vi "context.vi"(8 "error in (no error)":errorcluster) -> (0 "error out":errorcluster, 3 "Context Out":refnum<class "Context.lvclass">)   [LabVIEW 2019, in "Context.lvclass"]
doc: "This is a constructor VI, which builds, configures and returns a context to the calling code."
uses:
  Context.lvclass
  OOP States/Initialize References/Initialize References.lvclass
  C:/Users/fflores/Documents/GitHub Projects/Simon/Simon Game/OOP States/State/State.lvclass
  ContextData/ContextData.lvclass
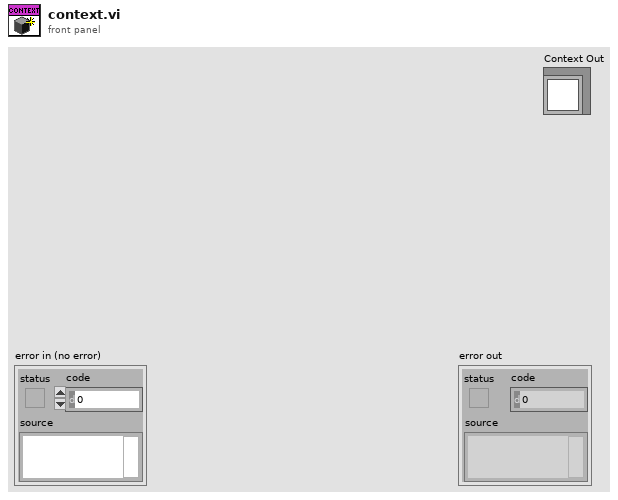
[diagram p1: front panel]
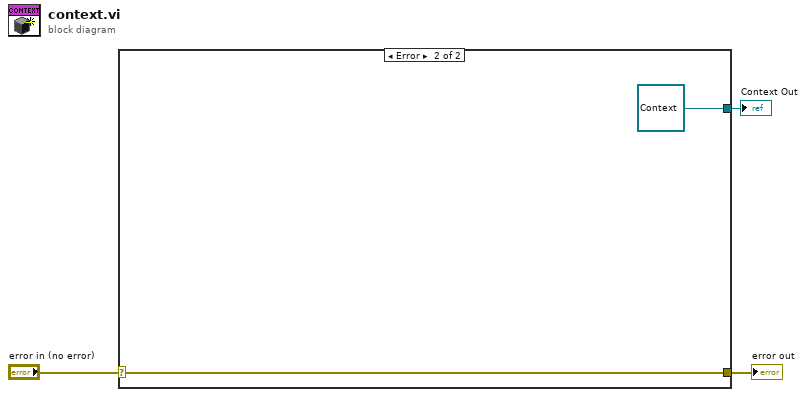
[diagram p0: block diagram]
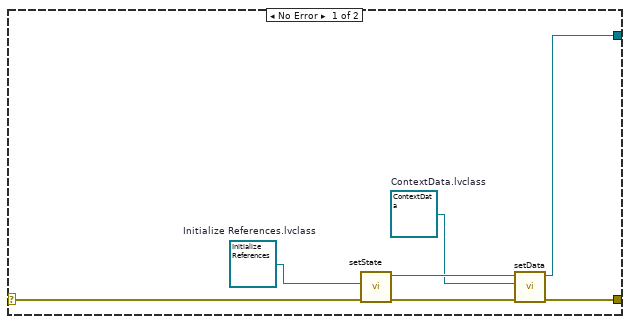
[diagram p2: hidden frame]
diagram:
  n1 = case shown="Error" "error in (no error)" {
    selector: "error in (no error)" -> [w10 w12]
    tunnel: [w7 w12] -> w2
    tunnel: [w4 refnum<class "Context.lvclass"> refnum ("Context.lvclass")] -> w1
    frame No Error {
      w5 = refnum<class "ContextData.lvclass"> refnum  # ContextData.lvclass
      w8 = refnum<class "Initialize References.lvclass"> refnum  # Initialize References.lvclass
      n2 = call "setState.vi"("error in (no error)"=w10, "State.lvclass"=w8) -> ("error out"=w9:errorcluster, "Context Out"=w6:refnum<class "Context.lvclass">)  [unwired: 8 in]
      n3 = call "setData.vi"("error in (no error)"=w9, "ContextData.lvclass"=w5, "Context In"=w6) -> ("error out"=w7:errorcluster, "Context Out"=w4:refnum<class "Context.lvclass">)  [unwired: 7 in]
    }
    frame Error {
    }
  }
  "error out" <- w2
  "Context Out" <- w1
